vi "Initialize.vi"(8 "error in (no error)":errorcluster, 9 "settings":T1, 10 "Transfer Groups Configurations":T2[](array[typedef]) {"Transfers"."channels"."string offset" format="%d bytes"}, 11 "Type Converter in":refnum<class "String Type Converter.lvclass">) -> (0 "error out":errorcluster, 3 "Type Converter out":refnum<class "String Type Converter.lvclass">)   [LabVIEW 2017, in "String Type Converter.lvlib" / "String Type Converter.lvclass"]
uses:
  String Type Converter.lvclass
  Builds/Data Sharing Framework/Current/Core/DSF Core.lvlibp/Typedefs/DSF Engine Transfer Group Configuration.ctl
  Builds/Data Sharing Framework/Current/Core/DSF Core.lvlibp/Typedefs/DSF Direction.ctl
  Builds/Data Sharing Framework/Current/Core/DSF Core.lvlibp/Typedefs/DSF Timing Info.ctl
  Builds/Data Sharing Framework/Current/Core/DSF Core.lvlibp/Typedefs/DSF Settings Info.ctl
  Builds/Data Sharing Framework/Current/Core/DSF Core.lvlibp/Typedefs/DSF Engine Transfer Configuration.ctl
  Builds/Data Sharing Framework/Current/Core/DSF Core.lvlibp/Typedefs/DSF Byte Order.ctl
  Builds/Data Sharing Framework/Current/Core/DSF Core.lvlibp/Typedefs/DSF Engine Channel Configuration.ctl
  Builds/Data Sharing Framework/Current/Core/DSF Core.lvlibp/Typedefs/DSF Data Type.ctl
  Builds/Data Sharing Framework/Current/Core/DSF Core.lvlibp/Typedefs/DSF Timeout Behavior.ctl
  Conversion.ctl
  Conversion Block.ctl
  String Type Converter.lvclass/String Type Converter.ctl
  Builds/Data Sharing Framework/Current/Core/DSF Core.lvlibp/Classes/Configuration/Required Buffer Size (Transfer Group).vi
  Builds/Data Sharing Framework/Current/Core/DSF Core.lvlibp
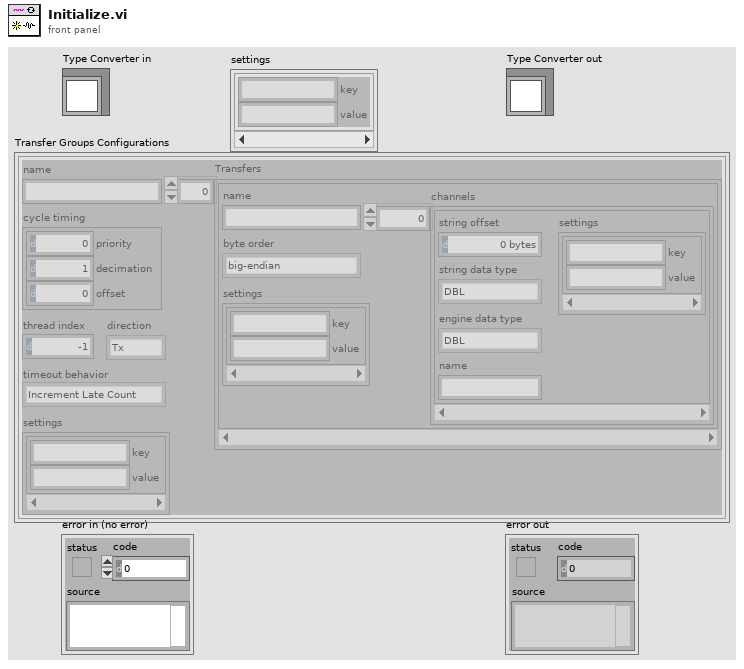
[diagram p1: front panel]
types:
  T1 = typedef "DSF Core.lvlibp/DSF Settings Info.ctl" = cluster{"key":string, "value":string}[]
  T2 = typedef "DSF Core.lvlibp/DSF Engine Transfer Group Configuration.ctl" = cluster{"name":string, "direction":T3, "cycle timing":T4, "thread index":i32, "settings":T1, "Transfers":T5[], "timeout behavior":T9}
  T3 = typedef "DSF Core.lvlibp/DSF Direction.ctl" = enum8{"Tx", "Rx"}
  T4 = typedef "DSF Core.lvlibp/DSF Timing Info.ctl" = cluster{"priority":u64, "decimation":u64, "offset":u64}
  T5 = typedef "DSF Core.lvlibp/DSF Engine Transfer Configuration.ctl" = cluster{"name":string, "byte order":T6, "settings":T1, "channels":T7[]}
  T6 = typedef "DSF Core.lvlibp/DSF Byte Order.ctl" = enum8{"big-endian", "little-endian"}
  T7 = typedef "DSF Core.lvlibp/DSF Engine Channel Configuration.ctl" = cluster{"string offset":u64, "string data type":T8, "engine data type":T8, "name":string, "settings":T1}
  T8 = typedef "DSF Core.lvlibp/DSF Data Type.ctl" = enum8{"Bool", "SGL", "DBL", "I8", "I16", "I32", "I64", "U8", "U16", "U32", "U64"}
  T9 = typedef "DSF Core.lvlibp/DSF Timeout Behavior.ctl" = enum8{"Increment Late Count", "Throw Error"}
  T10 = typedef "String Type Converter.lvlib/String Type Converter.lvclass/Conversion.ctl" = cluster{"conversion blocks":T11[]}
  T11 = typedef "String Type Converter.lvlib/String Type Converter.lvclass/Conversion Block.ctl" = cluster{"engine offset":u64, "engine data type":T8, "string offset":u64, "string data type":T8, "engine byte order":enum16{"big-endian, network order", "native, host order", "little-endian"}, "string byte order":enum16{"big-endian, network order", "native, host order", "little-endian"}, "count":u64}
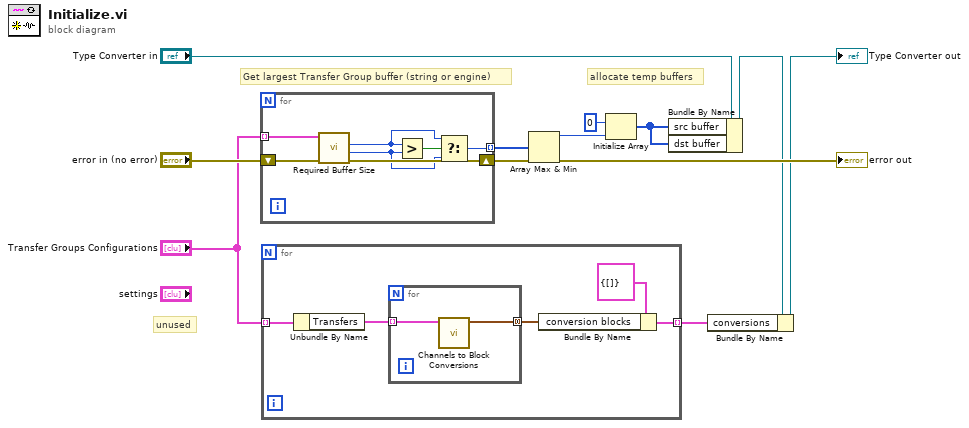
[diagram p0: block diagram]
diagram:
  # "Get largest Transfer Group buffer (string or engine)"
  # "unused"
  # "allocate temp buffers"
  n1 = for {
    tunnel: "Transfer Groups Configurations" -> [w17] mode=indexing
    tunnel: [w12] -> w10 mode=indexing
    shift-right: [w16] -> w11
    shift-left: "error in (no error)" -> [w18]
    n2 = call-poly "Required Buffer Size.vi"("error in (no error)"=w18, "Transfer Group Configuration in"=w17) -> ("error out"=w16:errorcluster, "total engine buffer size"=w13:u64, "total string buffer size"=w14:u64)  [unwired: 6 in, 1 out]
    n3 = Greater?(x=w14, y=w13) -> (0:w15:bool)
    n4 = Select(t=w14, s=w15, f=w13) -> (s? t:f=w12:u64)
  }
  "error out" <- w11
  n5 = for {
    tunnel: "Transfer Groups Configurations" -> [w22] mode=indexing
    tunnel: [w19] -> w6 mode=indexing
    n6 = Unbundle By Name(w22) -> ("Transfers"=w23:T5[])
    n7 = for {
      tunnel: w23 -> [w24] mode=indexing
      tunnel: [w25] -> w20 mode=concatenating
      n8 = call "Channels to Block Conversions.vi"("Transfer Configuration"=w24) -> ("Transfer conversion descriptors"=w25:T11[])  [unwired: 10 in]
    }
    n9 = Bundle By Name(cluster=T10 {"conversion blocks"=[]} ("conversion"), "conversion blocks"=w20) -> (w19:T10)
  }
  n10 = Array Max & Min(array=w10) -> (max value=w1:u64)  [unwired: 3 out]
  n11 = Initialize Array(u8 0 ("element"), w1) -> (w8:u8[])
  n12 = Bundle By Name(cluster="Type Converter in", "src buffer"=w8, "dst buffer"=w8) -> (w2:refnum<class "String Type Converter.lvclass">)
  n13 = Bundle By Name(cluster=w2, "conversions"=w6) -> (→"Type Converter out":refnum<class "String Type Converter.lvclass">)
